vi "F5xxx_get_scope_capabiilties.vi"(0 "sver":T1 caption="Scope version") -> (1 "has tunnel pulse":bool, 2 "has impedance":bool, 3 "has pulse period":bool)   [LabVIEW 2013]
uses:
  F5xxx_scope_type.ctl
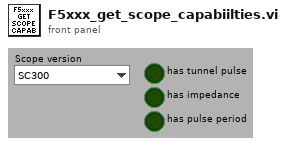
[diagram p1: front panel]
types:
  T1 = typedef "F5xxx_scope_type.ctl" = enum16{"SC300", "SC600/1100"}
  T2 = cluster{"tunnel pulse:":bool, "Z:":bool, "Pulse T:":bool}[]
  T3 = cluster{"tunnel pulse:":bool, "Z:":bool, "Pulse T:":bool}
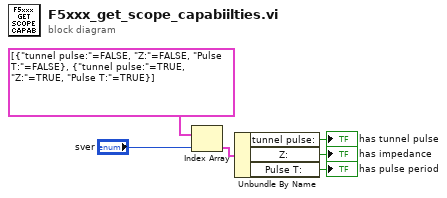
[diagram p0: block diagram]
diagram:
  n1 = Index Array(array=T2 [{"tunnel pulse:"=FALSE, "Z:"=FALSE, "Pulse T:"=FALSE}, {"tunnel pulse:"=TRUE, "Z:"=TRUE, "Pulse T:"=TRUE}], index="sver") -> (element=w4:T3)
  n2 = Unbundle By Name(w4) -> ("tunnel pulse:"=→"has tunnel pulse":bool, "Z:"=→"has impedance":bool, "Pulse T:"=→"has pulse period":bool)
